vi "Speed PID 3 motors.vi"(6 "dt (s)":dbl=0.02 format="%.3f", 7 "M Lift":dbl format="%#_4g", 8 "error in (no error)":errorcluster, 9 "PID gains":T1={"proportional gain (Kc)"=0.95, "integral time (Ti, min)"=0.01, "derivative time (Td, min)"=0.0} {"derivative time (Td, min)" format="%.3f"; "integral time (Ti, min)" format="%.3f"; "proportional gain (Kc)" format="%.3f"}, 10 "Motors Real":T2 {"M Real Lift" format="%#_4g"; "M Back" format="%#_4g"; "M Right" format="%#_4g"; "M Left" format="%#_4g"}, 11 "Motors":T3 {"M Back" format="%#_4g"; "M Right" format="%#_4g"; "M Left" format="%#_4g"}) -> (0 "error out":errorcluster, 3 "Motors Out":dbl[](array[numeric]) caption="输出" format="%.2f")   [LabVIEW 2020]
uses:
  <vilib>/addons/control/pid/pid.llb/PID (DBL).vi
  <vilib>/addons/control/pid/NI_PID_pid.lvlib
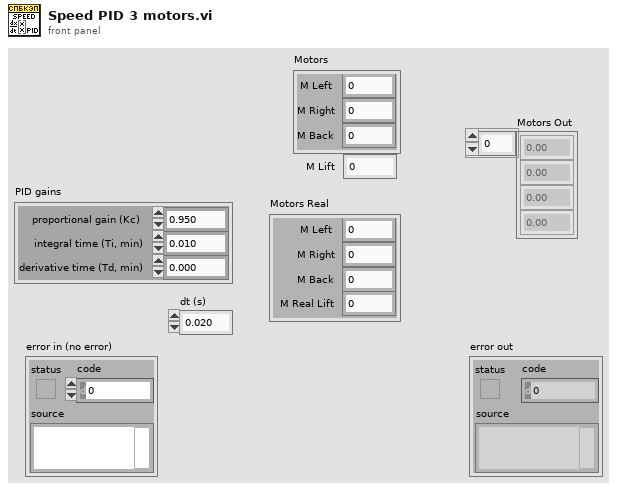
[diagram p1: front panel]
types:
  T1 = cluster{"proportional gain (Kc)":dbl, "integral time (Ti, min)":dbl, "derivative time (Td, min)":dbl}
  T2 = cluster{"M Left":dbl, "M Right":dbl, "M Back":dbl, "M Real Lift":dbl}
  T3 = cluster{"M Left":dbl, "M Right":dbl, "M Back":dbl}
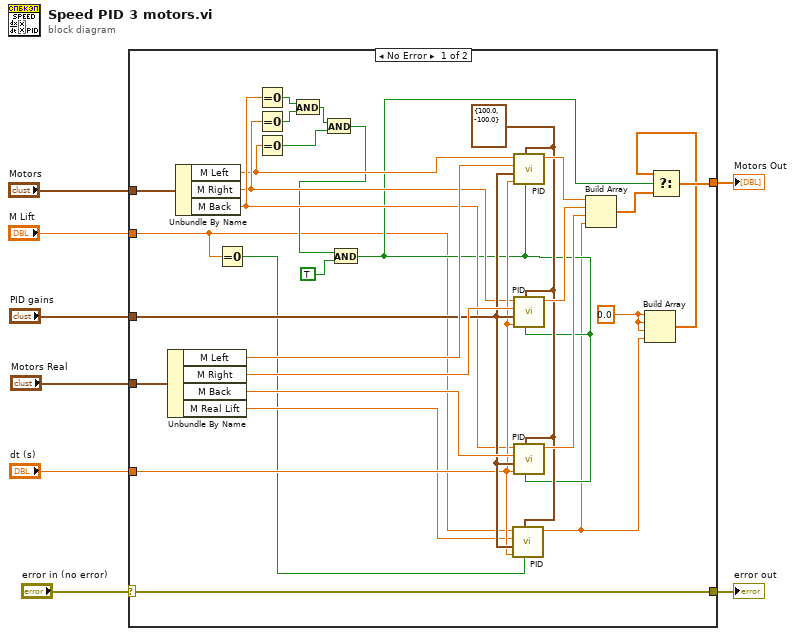
[diagram p0: block diagram]
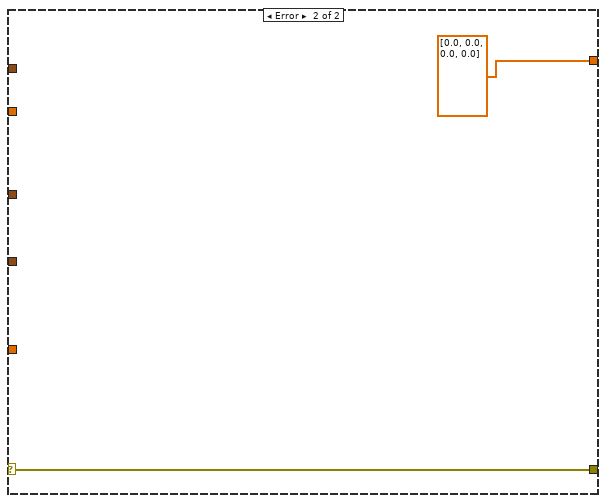
[diagram p2: hidden frame]
diagram:
  n1 = case shown="No Error" "error in (no error)" {
    selector: "error in (no error)" -> [w38 w40]
    tunnel: [w38 w40] -> w7
    tunnel: "dt (s)" -> [w27 _]
    tunnel: [w17 dbl[] [0.0, 0.0, 0.0, 0.0]] -> w5
    tunnel: "Motors" -> [w34 _]
    tunnel: "Motors Real" -> [w33 _]
    tunnel: "PID gains" -> [w28 _]
    tunnel: "M Lift" -> [w13 _]
    frame No Error {
      w11 = 0.0 ("element")
      w29 = cluster{"output high":dbl, "output low":dbl} {"output high"=100.0, "output low"=-100.0} ("output range")
      n2 = Unbundle By Name(w33) -> ("M Left"=w32:dbl, "M Right"=w31:dbl, "M Back"=w30:dbl, "M Real Lift"=w26:dbl)
      n3 = Unbundle By Name(w34) -> ("M Left"=w23:dbl, "M Right"=w24:dbl, "M Back"=w25:dbl)
      n4 = Equal To 0?(x=w13) -> (x = 0?=w12:bool)
      n5 = Equal To 0?(x=w25) -> (x = 0?=w22:bool)
      n6 = Equal To 0?(x=w24) -> (x = 0?=w21:bool)
      n7 = Equal To 0?(x=w23) -> (x = 0?=w19:bool)
      n8 = And(x=w22, y=w21) -> (x .and. y?=w20:bool)
      n9 = And(x=w20, y=w19) -> (x .and. y?=w16:bool)
      n10 = And(x=w16, y=TRUE) -> (x .and. y?=w14:bool)
      n11 = call-poly <vilib>:"PID.vi"("reinitialize? (F)"=w12, "output range"=w29, "dt (s)"=w27, "PID gains"=w28, "process variable"=w26, "setpoint"=w13) -> ("output"=w10:dbl)  [unwired: 4 in, 1 out]
      n12 = call-poly <vilib>:"PID.vi"("reinitialize? (F)"=w14, "output range"=w29, "dt (s)"=w27, "PID gains"=w28, "process variable"=w32, "setpoint"=w23) -> ("output"=w37:dbl)  [unwired: 4 in, 1 out]
      n13 = call-poly <vilib>:"PID.vi"("reinitialize? (F)"=w14, "output range"=w29, "dt (s)"=w27, "PID gains"=w28, "process variable"=w31, "setpoint"=w24) -> ("output"=w36:dbl)  [unwired: 4 in, 1 out]
      n14 = call-poly <vilib>:"PID.vi"("reinitialize? (F)"=w14, "output range"=w29, "dt (s)"=w27, "PID gains"=w28, "process variable"=w30, "setpoint"=w25) -> ("output"=w35:dbl)  [unwired: 4 in, 1 out]
      n15 = Build Array(w37, w36, w35, w10) -> (w18:dbl[])
      n16 = Build Array(w11, w11, w11, w10) -> (w9:dbl[])
      n17 = Select(t=w9, s=w14, f=w18) -> (s? t:f=w17:dbl[])
    }
    frame Error {
    }
  }
  "error out" <- w7
  "Motors Out" <- w5
